vi "Register gRPC Methods.vi"(8 "error in (no error)":errorcluster, 11 "Template Server in":refnum<class "OCVServer.lvclass">) -> (0 "error out":errorcluster, 3 "Template Server out":refnum<class "OCVServer.lvclass">)   [LabVIEW 2019, in "OCVServer.lvlib" / "OCVServer.lvclass"]
uses:
  OCVServer.lvclass
  typeDefs/Server Internal Message.ctl
  typeDefs/Server Internal Message UE.ctl
  typeDefs/Server Internal UEs.ctl
  gRPC lvSupport/Server API/typeDefs/grpcId.ctl
  gRPC lvSupport/gprc-lvsupport.lvlib
  gRPC lvSupport/Server API/typeDefs/gRPCId Cluster.ctl
  gRPC lvSupport/Server API/typeDefs/gRPCId Cluster UE.ctl
  typeDefs/Server gRPC UEs.ctl
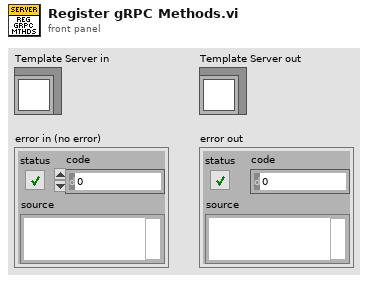
[diagram p1: front panel]
types:
  T1 = typedef "OCVServer.lvlib/OCVServer.lvclass/Server gRPC UEs.ctl" = cluster{"Template gRPCId UE":T2}
  T2 = typedef "OCVServer.lvlib/gprc-lvsupport.lvlib/gRPCId Cluster UE.ctl" = refnum<user-event>
  T3 = typedef "OCVServer.lvlib/OCVServer.lvclass/Server Internal UEs.ctl" = cluster{"Template Internal UE":T4}
  T4 = typedef "OCVServer.lvlib/OCVServer.lvclass/Server Internal Message UE.ctl" = refnum<user-event>
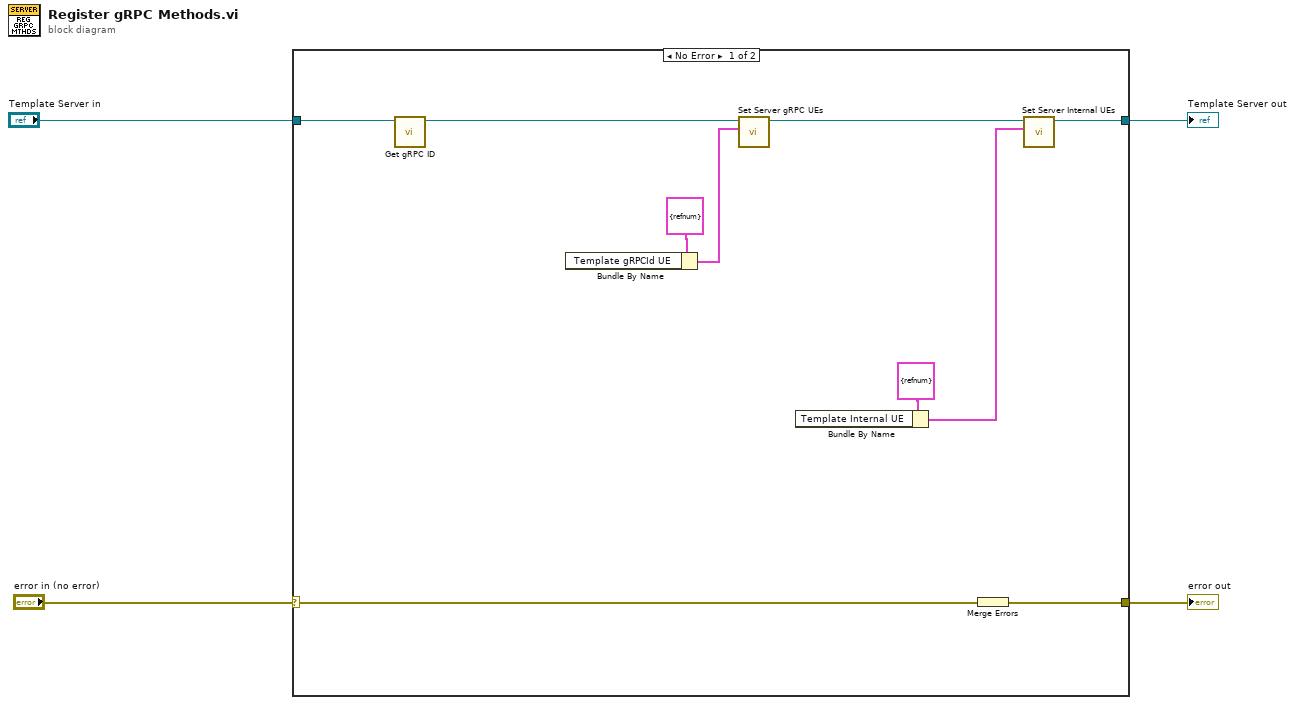
[diagram p0: block diagram]
diagram:
  n1 = case shown="No Error" "error in (no error)" {
    selector: "error in (no error)" -> [w5 w15]
    tunnel: "Template Server in" -> [w13 w16]
    tunnel: [w12 w15] -> w3
    tunnel: [w11 w16] -> w2
    frame No Error {
      n2 = call "Get gRPC ID.vi"("OOP Server in"=w13) -> ("OOP Server out"=w14:refnum<class "OCVServer.lvclass">)  [unwired: 9 in, 1 out]
      n3 = Bundle By Name ("Bundle gRPC UEs")(cluster=T1 {"Template gRPCId UE"=refnum} ("gRPC Server Method Events")) -> (w7:T1)  [unwired: 1 in]
      n4 = call "Set Server gRPC UEs.vi"("Server gRPC UEs"=w7, "OOP Server in"=w14) -> ("OOP Server out"=w8:refnum<class "OCVServer.lvclass">)  [unwired: 9 in]
      n5 = Bundle By Name ("Bundle Internal UEs")(cluster=T3 {"Template Internal UE"=refnum} ("Server Internal UEs")) -> (w10:T3)  [unwired: 1 in]
      n6 = Merge Errors(w5) -> (w12:errorcluster)
      n7 = call "Set Server Internal UEs.vi"("Server Internal UEs"=w10, "OOP Server in"=w8) -> ("OOP Server out"=w11:refnum<class "OCVServer.lvclass">)  [unwired: 9 in]
    }
    frame Error {
    }
  }
  "error out" <- w3
  "Template Server out" <- w2
